vi "Digital DAQ Configure.vi"(8 "error in":errorcluster, 10 "Port Digitales":tag[](array[tag]), 11 "DAQmx Device Digital":tag) -> (0 "error out":errorcluster, 3 "task out":refnum<k21>)   [LabVIEW 2020]
uses:
  <vilib>/DAQmx/create/channels.llb/DAQmx Create Channel (DI-Digital Input).vi
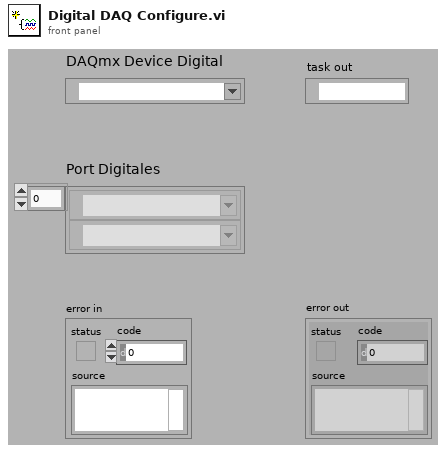
[diagram p1: front panel]
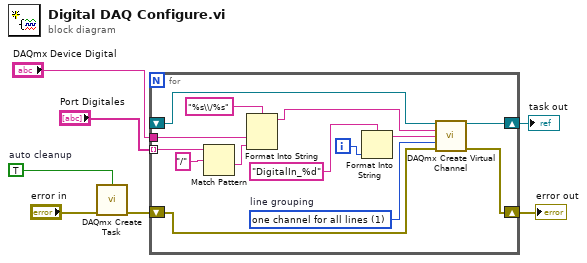
[diagram p0: block diagram]
diagram:
  w4 = TRUE  # auto cleanup
  n1 = call <vilib>:"DAQmx Create Task.vi"("auto cleanup"=w4, "error in"="error in") -> ("error out"=w2:errorcluster)  [unwired: 12 in, 1 out]
  n2 = for {
    shift-right: [w13] -> w7
    shift-left: w2 -> [w8]
    shift-right: [w14] -> w1
    shift-left: _ -> [w12]
    tunnel: "Port Digitales" -> [w17] mode=indexing
    tunnel: "DAQmx Device Digital" -> [w21]
    i -> [w16]
    w9 = 1 items=["one channel for each line", "one channel for all lines"]  # line grouping
    n3 = Match Pattern(string=w17, regular expression="/") -> (after substring=w20:string)  [unwired: 1 in, 3 out]
    n4 = Format Into String(format string="%s\\/%s", w21, w20) -> (resulting string=w11:string)  [unwired: 2 in, 1 out]
    n5 = Format Into String(format string="DigitalIn_%d", w16) -> (resulting string=w10:string)  [unwired: 2 in, 1 out]
    n6 = call-poly <vilib>:"DAQmx Create Virtual Channel.vi"("task in"=w12, "lines"=w11, "name to assign"=w10, "line grouping"=w9, "error in"=w8) -> ("task out"=w14:refnum<k21>, "error out"=w13:errorcluster)  [unwired: 9 in]
  }
  "error out" <- w7
  "task out" <- w1
